vi "Add Child Items to Tree.vi"(8 "error in":errorcluster, 10 "Dynamic Dispatch VI Type in":refnum<class "Dynamic Dispatch VI Type.lvclass">, 11 "Tree Ref in":refnum<vi>) -> (0 "error out":errorcluster, 2 "Dynamic Dispatch VI Type out":refnum<class "Dynamic Dispatch VI Type.lvclass">, 3 "Tree Ref out":refnum<vi>)   [LabVIEW 2020, in "Peek Window.lvlib" / "Dynamic Dispatch VI Type.lvclass"]
uses:
  Dynamic Dispatch VI Type.lvclass
  D:/Code/VI-Peek/source/Peek Window/VI Types/Standard VI Type/Standard VI Type.lvclass
  Symbols Enum.ctl
  Dynamic Dispatch VI Type.lvclass/Dynamic Dispatch VI Type.ctl
  Standard VI Type/Standard VI Type.lvclass/Standard VI Type.ctl
  Standard VI Type/Read Selectable.vi
  Standard VI Type/Read Full Qualified Name.vi
  Implementation VI Type/Implementation VI Type.lvclass
  Peek Window.lvlib
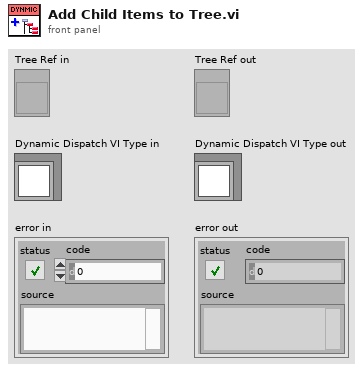
[diagram p1: front panel]
types:
  T1 = typedef "Peek Window.lvlib/Symbols Enum.ctl" = enum16{"<Blank>", "Below Here Glyph", "VI", "Dynamic Dispatch VI", "Malleable VI", "Polymorphic VI", "Missing VI", "Express VI"}
  T2 = map{string, refnum<class "Implementation VI Type.lvclass">}
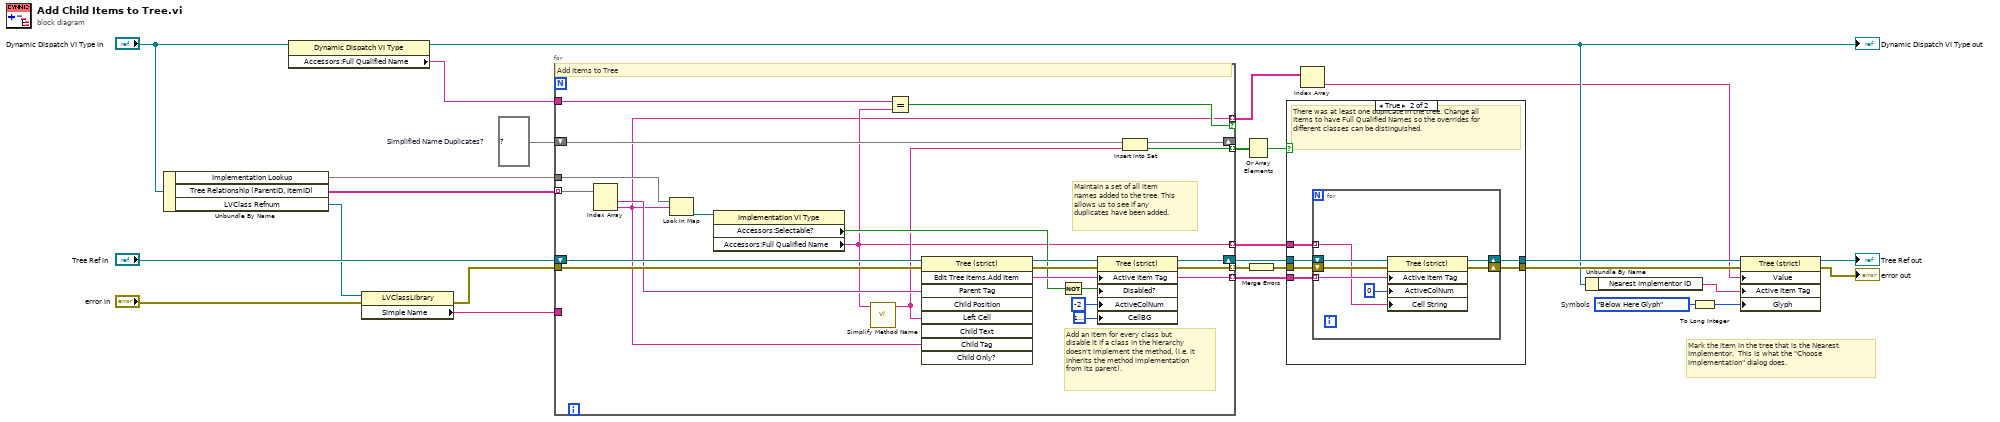
[diagram p0: block diagram]
diagram:
  w13 = Symbols_Enum."Below Here Glyph"  # Symbols
  w12 = set{string} {}  # Simplified Name Duplicates?
  # "Mark the item in the tree that is the Nearest Implementor.  This is what the \"Choose Implementation\" dialog does."
  n1 = Unbundle By Name("Dynamic Dispatch VI Type in") -> ("Implementation Lookup"=w18:T2, "Tree Relationship (ParentID, ItemID)"=w19:string[][], "LVClass Refnum"=w5:refnum<vi>)
  n2 = property class="Dynamic Dispatch VI Type"(reference="Dynamic Dispatch VI Type in") -> (reference out=w4:refnum<class "Dynamic Dispatch VI Type.lvclass">, "Accessors:Full Qualified Name"=w3:string)  [unwired: 1 in, 1 out]
  "Dynamic Dispatch VI Type out" <- w4
  n3 = property class="LVClassLibrary"(reference=w5, error in="error in") -> (error out=w20:errorcluster, "Simple Name"=w21:string)  [unwired: 1 out]
  n4 = for {
    tunnel: [w49] -> w10 mode=indexing
    tunnel: [w30] -> w11 mode=indexing
    tunnel: [w46] -> w7 mode=indexing
    shift-right: [w47] -> _
    shift-left: w12 -> [w48]
    shift-right: [w50] -> w9
    shift-left: "Tree Ref in" -> [w45]
    tunnel: w19 -> [w43] mode=indexing
    tunnel: w20 -> [w41]
    tunnel: w21 -> [_]
    tunnel: [w39] -> w22 mode=indexing
    tunnel: w18 -> [w44]
    tunnel: w3 -> [w31]
    tunnel: [w28] -> w2 mode=indexing if=w29
    # "Add an item for every class but disable it if a class in the hierarchy doesn't implement the method, (i.e. it inherits the method implementation from its parent)."
    # "Maintain a set of all item names added to the tree. This allows us to see if any duplicates have been added."
    # "Add Items to Tree"
    n5 = Index Array(array=w43) -> (element #1=w40:string, element #2=w28:string)  [unwired: 2 in]
    n6 = Look In Map(map=w44, key=w28) -> (value=w42:refnum<class "Implementation VI Type.lvclass">)  [unwired: 1 in, 1 out]
    n7 = property class="Implementation VI Type"(reference=w42) -> ("Accessors:Selectable?"=w34:bool, "Accessors:Full Qualified Name"=w30:string)  [unwired: 1 in, 2 out]
    n8 = call "Simplify Method Name.vi"("Method Full Qualified Name"=w30) -> ("Class and Method Only"=w33:string)  [unwired: 10 in]
    n9 = Equal?(x=w31, y=w30) -> (x = y?=w29:bool)
    n10 = invoke class="Tree (strict)" method="Edit Tree Items.Add Item"(reference=w45, error in=w41, "Parent Tag"=w40, "Left Cell"=w33, "Child Tag"=w28) -> (reference out=w38:refnum<vi>, error out=w37:errorcluster, "Edit Tree Items:Add Item"=w49:string)  [unwired: 4 in, 6 out]
    n11 = Not(x=w34) -> (.not. x?=w36:bool)
    n12 = property class="Tree (strict)"(reference=w38, error in=w37, "Active Item Tag"=w49, "Disabled?"=w36, "ActiveColNum"=-2, "CellBG"=u32 16777238) -> (reference out=w50:refnum<vi>, error out=w39:errorcluster)
    n13 = Insert Into Set(10:w33, 11:w48) -> (2:w46:bool, 3:w47:set{string})
  }
  n14 = Or Array Elements(Boolean array=w7) -> (logical OR=w8:bool)
  n15 = Merge Errors(w22) -> (w23:errorcluster)
  n16 = case shown="True" w8 {
    tunnel: w9 -> [w52 w56]
    tunnel: [w52 w55] -> w14
    tunnel: w23 -> [w51 w54]
    tunnel: [w51 w53] -> w16
    tunnel: w10 -> [_ w58]
    tunnel: w11 -> [_ w57]
    frame False {
      # "No duplicate items in the tree, no need to update class file names in the tree to qualified class names."
    }
    frame True {
      # "There was at least one duplicate in the tree. Change all items to have Full Qualified Names so the overrides for different classes can be distinguished."
      n17 = for {
        tunnel: w58 -> [w61] mode=indexing
        tunnel: w57 -> [w59] mode=indexing
        shift-right: [w64] -> w55
        shift-left: w56 -> [w65]
        shift-right: [w62] -> w53
        shift-left: w54 -> [w63]
        n18 = property class="Tree (strict)"(reference=w65, error in=w63, "Active Item Tag"=w61, "ActiveColNum"=0 ("Active Cell:Active Column Number"), "Cell String"=w59) -> (reference out=w64:refnum<vi>, error out=w62:errorcluster)
      }
    }
  }
  n19 = Index Array(array=w2) -> (element=w1:string)  [unwired: 1 in]
  n20 = Unbundle By Name(w4) -> ("Nearest Implementor ID"=w17:string)
  n21 = To Long Integer(number=w13) -> (32bit integer=w15:i32)
  n22 = property class="Tree (strict)"(reference=w14, error in=w16, "Value"=w1, "Active Item Tag"=w17, "Glyph"=w15) -> (reference out=→"Tree Ref out":refnum<vi>, error out=→"error out":errorcluster)
